vi "RECV.vi"(8 "error in (no error)":errorcluster, 9 "timeout ms (100)":i32=100, 11 "connection ID":refnum<k5>) -> (0 "error out":errorcluster, 1 "msg recv'd?":bool, 2 "recv data":string, 3 "connection ID out":refnum<k5>)   [LabVIEW 2023]
panel:
  out "bytes to follow":i32
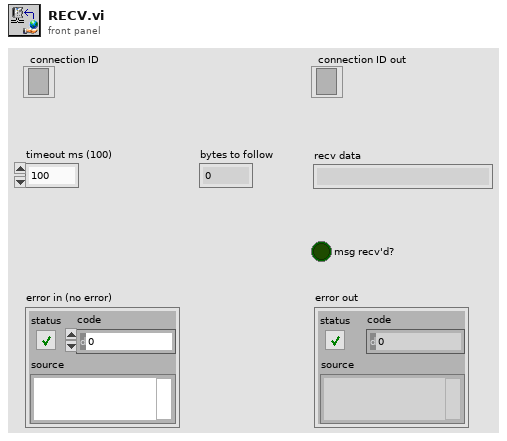
[diagram p1: front panel]
types:
  T1 = enum16{"Standard", "Buffered", "CRLF", "Immediate"}
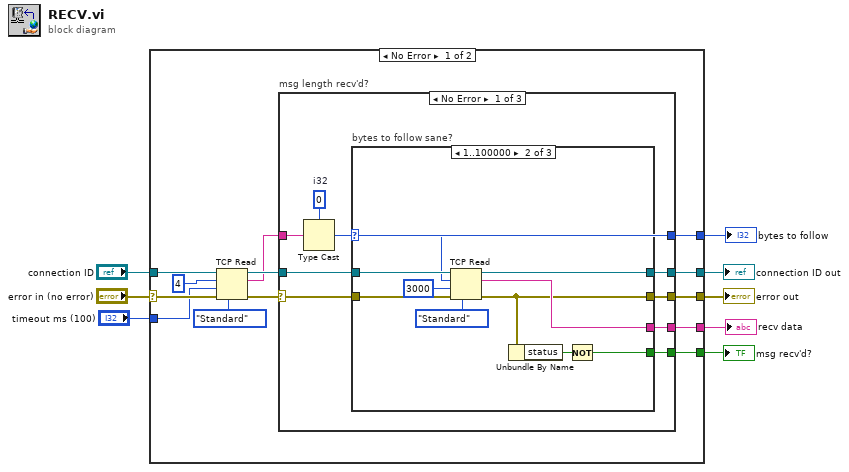
[diagram p0: block diagram]
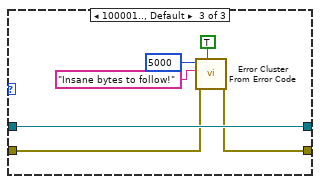
[diagram p3: hidden frame]
diagram:
  n1 = case shown="No Error" "error in (no error)" {
    selector: "error in (no error)" -> [w20 w52]
    tunnel: "connection ID" -> [w21 w53]
    tunnel: [w14 w53] -> w7
    tunnel: [w16 w52] -> w6
    tunnel: [w12 _] -> w4
    tunnel: [w11 _] -> w3
    tunnel: "timeout ms (100)" -> [w10 _]
    tunnel: [w9 _] -> w1
    frame No Error {
      n2 = TCP Read(connection ID=w21, bytes to read=4, error in (no error)=w20, 7:T1."Standard" ("mode (standard)"), 9:w10) -> (connection ID out=w15:refnum<k5>, data out=w13:string, error out=w17:errorcluster)
      n3 = case "msg length recv'd?" shown="No Error" w17 {
        selector: w17 -> [w29 w50 _]
        tunnel: [w24 w50 _] -> w16
        tunnel: w15 -> [w30 w49 w51]
        tunnel: [w28 w49 w51] -> w14
        tunnel: w13 -> [w26 _ _]
        tunnel: [w27 _ _] -> w12
        tunnel: [w22 _ _] -> w11
        tunnel: [w23 _ _] -> w9
        frame No Error {
          w25 = 0  # i32
          n4 = Type Cast(type=w25, x=w26) -> (*(type *) &x=w22:i32)
          n5 = case "bytes to follow sane?" shown="1..100000" w22 {
            selector: w22 -> [_ w33 _]
            tunnel: w30 -> [w32 w42 w48]
            tunnel: w29 -> [w31 w41 w46]
            tunnel: [w32 w40 w48] -> w28
            tunnel: [_ w39 _] -> w27
            tunnel: [w31 w36 w45] -> w24
            tunnel: [_ w34 _] -> w23
            frame 0 {
            }
            frame 1..100000 {
              n6 = TCP Read(connection ID=w42, bytes to read=w33, error in (no error)=w41, 7:T1."Standard" ("mode (standard)"), 9:3000 ("timeout ms (25000)")) -> (connection ID out=w40:refnum<k5>, data out=w39:string, error out=w36:errorcluster)
              n7 = Unbundle By Name(w36) -> ("status"=w35:bool)
              n8 = Not(x=w35) -> (.not. x?=w34:bool)
            }
            frame 100001.., Default {
              n9 = call <vilib>:"Error Cluster From Error Code.vi"("show call chain? (False)"=TRUE, "error in (no error)"=w46, "error message (\"\")"="Insane bytes to follow!" ("source"), "error code (0)"=5000 ("code")) -> ("error out"=w45:errorcluster)  [unwired: 5 in]
            }
          }
        }
        frame Default {
        }
        frame Error {
          # "recv timed out, no msg pending\nclear and move on"
        }
      }
    }
    frame Error {
    }
  }
  "error out" <- w6
  "recv data" <- w4
  "connection ID out" <- w7
  "bytes to follow" <- w3
  "msg recv'd?" <- w1
